vi "SPI_GetChipSelectActiveState.vi"(5 "Device":i32, 7 "Bus":i32=1, 8 "error in":errorcluster) -> (0 "error out":errorcluster, 4 "CS active state":bool)   [LabVIEW 2014, in "GPIO.lvlib"]
doc: "Reads the active state of the Chip Select pin for the specified SPI device."
uses:
  GPIO.lvlib
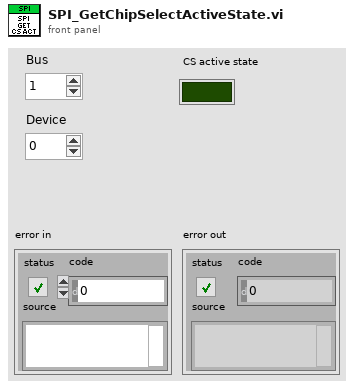
[diagram p1: front panel]
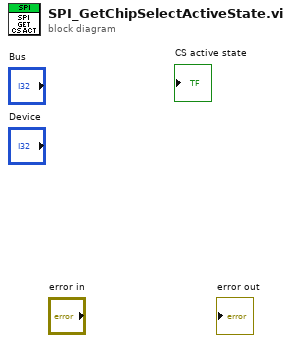
[diagram p0: block diagram]
diagram:
